vi "CAN_Reset.vi"(8 "错误输入（无错误）":errorcluster, 11 "General_Input":T2) -> (0 "错误输出":errorcluster, 2 "Reset":bool, 3 "General_Output":T1)   [LabVIEW 2012]
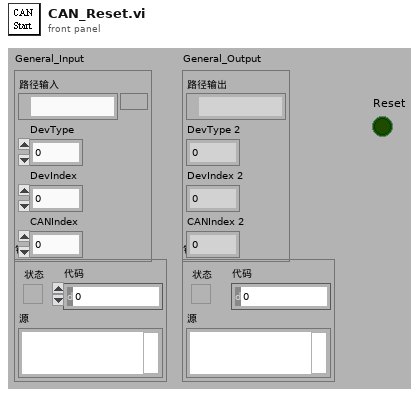
[diagram p1: front panel]
types:
  T1 = cluster{"路径输出":path, "DevType 2":u32, "DevIndex 2":u32, "CANIndex 2":u32}
  T2 = cluster{"路径输入":path, "DevType":u32, "DevIndex":u32, "CANIndex":u32}
  T3 = cluster{"path out":path, "DevType":u32, "DevIndex":u32, "CANIndex":u32}
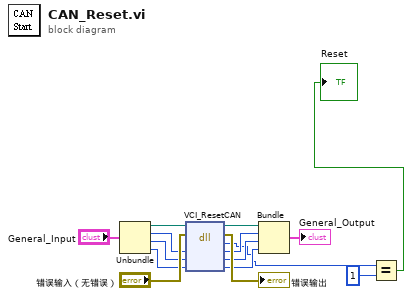
[diagram p0: block diagram]
diagram:
  n1 = Unbundle("General_Input") -> ("路径输入"=w12:path, "DevType"=w9:u32, "DevIndex"=w10:u32, "CANIndex"=w11:u32)
  n2 = dll-call lib="PTH1babs CUsershantt.GLBPOWERDesktop殷浩485双串口_20130710_01USBCAN2ControlCAN.dll" fn="VCI_ResetCAN" ("ControlCAN.dll:VCI_StartCAN")(path in=w12, error in="错误输入（无错误）", "DevType"=w9, "DevIndex"=w10, "CANIndex"=w11) -> (path out=w8:path, error out=→"错误输出":errorcluster, "返回类型"=w3:u32, "DevType"=w5:u32, "DevIndex"=w6:u32, "CANIndex"=w7:u32)  [unwired: 1 in]
  n3 = Bundle("path out"=w8, "DevType"=w5, "DevIndex"=w6, "CANIndex"=w7) -> (→"General_Output":T3)  [unwired: 1 in]
  n4 = Equal?(x=w3, y=u32 1) -> (x = y?=→"Reset":bool)
